vi "Init.vi"(8 "error in (no error)":errorcluster, 9 "Configuration File Path":path=path "", 10 "Process Name":string, 11 "Error Handler In":refnum<class "Error Handler.lvclass">) -> (0 "error out":errorcluster, 3 "Error Handler Out":refnum<class "Error Handler.lvclass">)   [LabVIEW 2020, in "Error Handler.lvclass"]
uses:
  Error Handler.lvclass
  Public/TypeDefs/Error Message Data.ctl
  Process/Process.lvclass
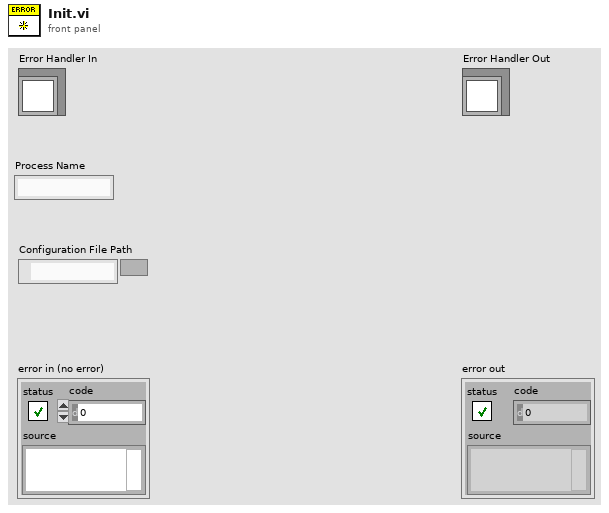
[diagram p1: front panel]
types:
  T1 = typedef "Error Handler.lvclass/Error Message Data.ctl" = cluster{"Error Type":string, "Location":string, "Error":errorcluster}
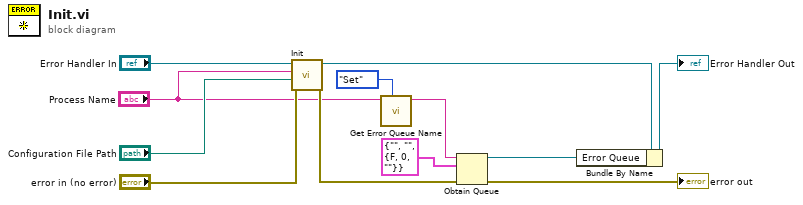
[diagram p0: block diagram]
diagram:
  n1 = call-parent "Init.vi"("error in (no error)"="error in (no error)", "Config File Path"="Configuration File Path", "Name"="Process Name", "Process In"="Error Handler In") -> ("error out"=w6:errorcluster, "Process Out"=w12:refnum<class "Error Handler.lvclass">)  [unwired: 6 in]
  n2 = call "Get Error Queue Name.vi"("Action"=enum16{"Get", "Set"}."Set", "Queue Name"="Process Name") -> ("Queue Name"=w7:string)  [unwired: 8 in, 1 out]
  n3 = Obtain Queue(name (unnamed)=w7, element data type=T1 {"Error Type"="", "Location"="", "Error"={"status"=FALSE, "code"=0, "source"=""}} ("Error Message Data"), error in (no error)=w6) -> (queue out=w5:refnum<queue>, error out=→"error out":errorcluster)  [unwired: 2 in, 1 out]
  n4 = Bundle By Name(cluster=w12, "Error Queue"=w5) -> (→"Error Handler Out":refnum<class "Error Handler.lvclass">)
